vi "TcpProtocoalUnderstandingServerSide.vi"() -> ()   [LabVIEW 2019]
panel:
  in  "stop":bool
  out "offset past number":i32
  in  "bytes to read":i32
  in  "mode (standard) 2":T1(ring)
  out "Thermometer":dbl(slide) scale=0.0..100.0
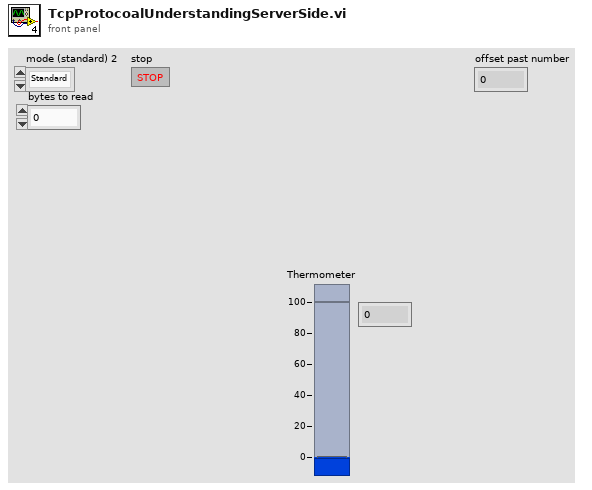
[diagram p1: front panel]
types:
  T1 = enum16{"Standard", "Buffered", "CRLF", "Immediate"}
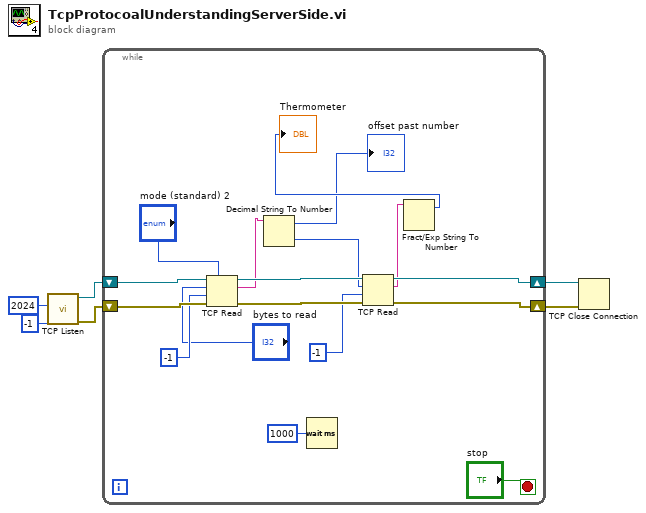
[diagram p0: block diagram]
diagram:
  n1 = call <vilib>:"TCP Listen.vi"("timeout ms (wait forever: -1)"=-1, "port"=u16 2024) -> ("error out"=w2:errorcluster, "connection ID"=w4:refnum<k5>)  [unwired: 5 in, 3 out]
  n2 = while {
    shift-right: [w21] -> w3
    shift-left: w4 -> [w23]
    shift-right: [w18] -> w1
    shift-left: w2 -> [w20]
    stop <- "stop" stop-if-true
    n3 = TCP Read(connection ID=w23, bytes to read="bytes to read", error in (no error)=w20, 7:"mode (standard) 2", 9:-1 ("timeout ms (25000)")) -> (connection ID out=w22:refnum<k5>, data out=w12:string, error out=w19:errorcluster)
    n4 = Decimal String To Number(string=w12) -> (offset past number=→"offset past number":i32, number=w11:i32)  [unwired: 2 in]
    n5 = Wait (ms)(milliseconds to wait=u32 1000) -> ()  [unwired: 1 out]
    n6 = TCP Read(connection ID=w22, bytes to read=w11, error in (no error)=w19, 9:-1 ("timeout ms (25000)")) -> (connection ID out=w21:refnum<k5>, data out=w13:string, error out=w18:errorcluster)  [unwired: 1 in]
    n7 = Fract/Exp String To Number(string=w13) -> (offset past number=→"Thermometer":i32)  [unwired: 3 in, 1 out]
  }
  n8 = TCP Close Connection(connection ID=w3, error in (no error)=w1) -> ()  [unwired: 1 in, 2 out]
